vi "Release.vi"(8 "Error In":errorcluster, 11 "Bool In":refnum<class "Bool.lvclass">) -> (0 "Error Out":errorcluster)   [LabVIEW 2016, in "Bool.lvclass"]
uses:
  Bool.lvclass
  Tree Data/Tree Data.lvclass
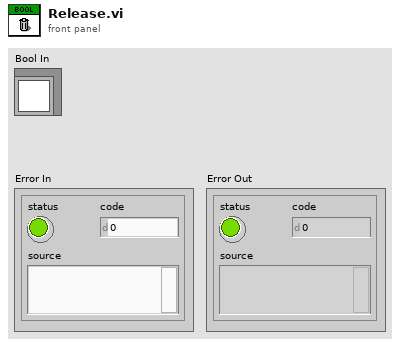
[diagram p1: front panel]
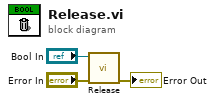
[diagram p0: block diagram]
diagram:
  n1 = call-parent "Release.vi"("Error In"="Error In", "Tree Data In"="Bool In") -> ("Error Out"=→"Error Out":errorcluster)  [unwired: 9 in]
